vi "moving_average_filter.vi"(1 "Maximum Window":i32=5, 2 "X":dbl) -> (0 "Filtered x":dbl)   [LabVIEW 2023]
panel:
  out "Counter":dbl=1.0
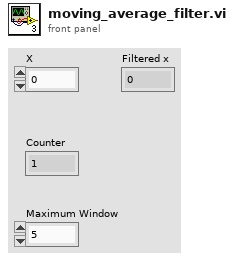
[diagram p1: front panel]
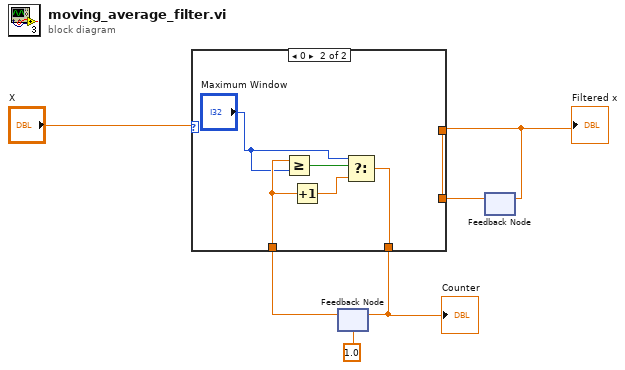
[diagram p0: block diagram]
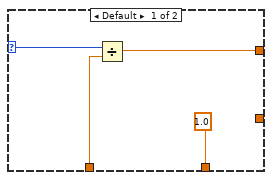
[diagram p2: hidden frame]
diagram:
  n1 = feedback #1(1.0) -> (w2:dbl)
  n2 = feedback #2() -> (w4:dbl)  [unwired: 1 in]
  n3 = case shown="0" "X" {
    selector: "X" -> [w10 _]
    tunnel: [w9 w16] -> w5
    tunnel: w4 -> [_ w16]
    tunnel: [1.0 w12] -> w3
    tunnel: w2 -> [w7 w13]
    frame Default {
      n4 = Divide(x=w10, y=w7) -> (x/y=w9:dbl)
    }
    frame 0 {
      n5 = Greater Or Equal?(x=w13, y="Maximum Window") -> (x >= y?=w15:bool)
      n6 = Increment(x=w13) -> (x+1=w14:dbl)
      n7 = Select(t="Maximum Window", s=w15, f=w14) -> (s? t:f=w12:dbl)
    }
  }
  "Filtered x" <- w5
  "Counter" <- w3
  n8 = feedback-in #1(w3) -> ()
  n9 = feedback-in #2(w5) -> ()
